vi "AddName.vi"() -> (2 "Cancel Indicator":bool, 3 "NameString":string)   [LabVIEW 2013, in "main.lvlib"]
uses:
  main.lvlib
panel:
  out "AddName_TitleString":string
  in  "AddName_CancelBtn":bool caption="CancelBtn"
  in  "AddName_SaveBtn":bool caption="SaveBtn"
  in  "AddName_Name":string caption="Name"
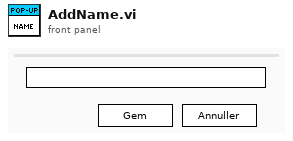
[diagram p1: front panel]
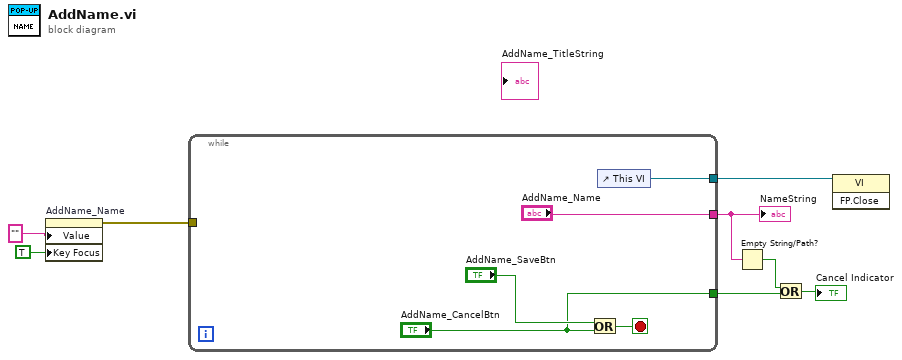
[diagram p0: block diagram]
diagram:
  n1 = property on="AddName_Name" class="Str"("Value"="" ("Name"), "Key Focus"=TRUE) -> (error out=w6:errorcluster)  [unwired: 2 in, 1 out]
  n2 = while {
    tunnel: [w11] -> w8
    tunnel: w6 -> [_]
    tunnel: ["AddName_Name"] -> w4
    tunnel: ["AddName_CancelBtn"] -> w1
    stop <- w12 stop-if-true
    n3 = Or(x="AddName_SaveBtn", y="AddName_CancelBtn") -> (x .or. y?=w12:bool)
    n4 = control-ref of="This VI"() -> (w11:refnum<vi>)
  }
  "NameString" <- w4
  n5 = Empty String/Path?(string/path=w4) -> (empty?=w2:bool)
  n6 = Or(x=w2, y=w1) -> (x .or. y?=→"Cancel Indicator":bool)
  n7 = invoke class="VI" method="FP.Close"(reference=w8) -> ()  [unwired: 2 in, 3 out]
